vi "delete0.vi"(10 "Array In":dbl[](array[numeric]), 11 "Storage Array in":dbl[](array[numeric])) -> (3 "Storage Array out":dbl[](array[numeric]))   [LabVIEW 2013]
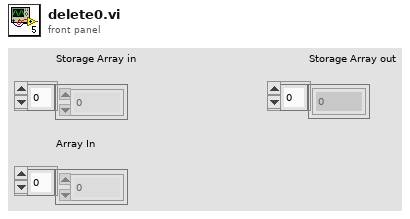
[diagram p1: front panel]
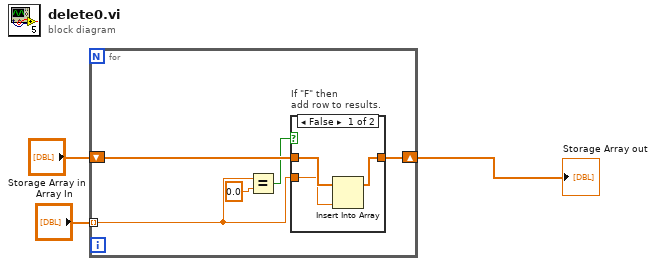
[diagram p0: block diagram]
diagram:
  n1 = for {
    tunnel: "Array In" -> [w6] mode=indexing
    shift-right: [w7] -> w3
    shift-left: "Storage Array in" -> [w8]
    n2 = Equal?(x=w6, y=0.0) -> (x = y?=w4:bool)
    n3 = case "If \"F\" then \nadd row to results." shown="False" w4 {
      tunnel: w8 -> [w11 w12]
      tunnel: w6 -> [w10 _]
      tunnel: [w9 w12] -> w7
      frame False {
        n4 = Insert Into Array(array=w11, new element=w10) -> (w9:dbl[])  [unwired: 1 in]
      }
      frame True {
      }
    }
  }
  "Storage Array out" <- w3
